vi "Receive Command.vi"(10 "Consumer Queues":T1, 11 "Generic Command in":refnum<class "Generic Command.lvclass">) -> (0 "error out":errorcluster, 3 "Generic Command out":refnum<class "Generic Command.lvclass">)   [LabVIEW 2019, in "Generic Command.lvclass"]
uses:
  Generic Command.lvclass
  TS Framework/Consumer Queues.ctl
  UI Process/Generic UI Command/Generic UI Process Command.lvclass
  DAC Process/Generic DAC Command/Generic DAC Process Command.lvclass
  Trig Process/Generic Trig Command/Generic Trig Process Command.lvclass
  TS Framework/TS Framework.lvlib
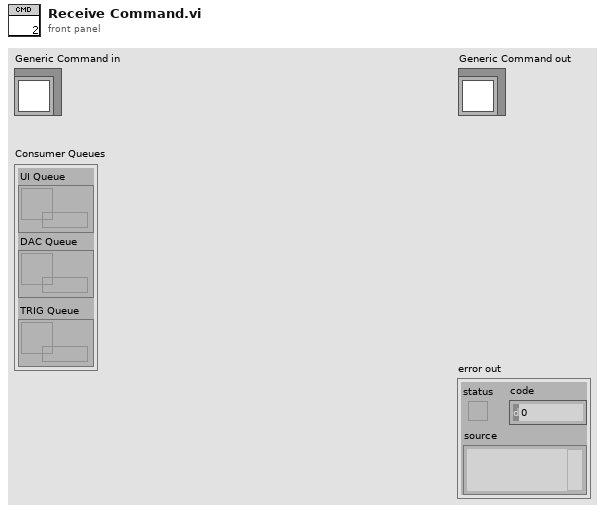
[diagram p1: front panel]
types:
  T1 = typedef "TS Framework.lvlib/Consumer Queues.ctl" = cluster{"UI Queue":refnum<queue>, "DAC Queue":refnum<queue>, "TRIG Queue":refnum<queue>}
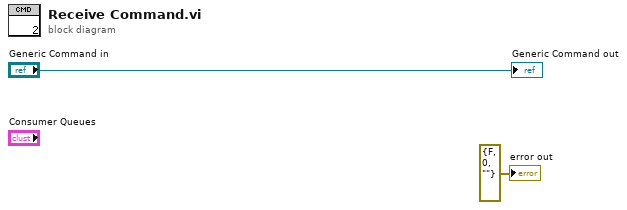
[diagram p0: block diagram]
diagram:
  "error out" <- errorcluster {"status"=FALSE, "code"=0, "source"=""} ("error out")
  "Generic Command out" <- "Generic Command in"
